vi "禹山pH校准.vi"() -> ()   [LabVIEW 2016, in "斯坦道多参数.lvlib"]
uses:
  <vilib>/Utility/miscctls.llb/LVPointTypeDef.ctl
  <vilib>/Analysis/NI_AALBase.lvlib
  <vilib>/Analysis/NI_AALPro.lvlib
  <vilib>/Utility/config.llb/NI_LVConfig.lvlib
panel:
  out "通讯状态":string
  out "第二点校准值":dbl
  out "第一点校准值":dbl
  out "最小值":sgl format="%.2g"
  out "最大值":sgl format="%.2g"
  in  "校准停止":bool
  in  "校准模式":u16(ring) items=["两点校准", "单点校准"]
  in  "标液2":dbl
  in  "标液1":dbl
  out "波形图表":sgl(graph) caption="历史曲线"
  out "温度测量值":dbl caption="温度" format="%#.2f"
  out "变异系数":dbl format="%.6g"
  out "standard deviation":dbl caption="标准差" format="%0.2f"
  out "mean":dbl caption="均值" format="%0.2f"
  out "提示":string
  in  "校准启动":bool
  out "测试值":dbl format="%#.2f"
  out "电极斜率":dbl format="%#.6f"
  out "电极零点":dbl format="%#.6f"
  # "酸碱度电极设定"
  # "℃"
  # "请选择校准模式:"
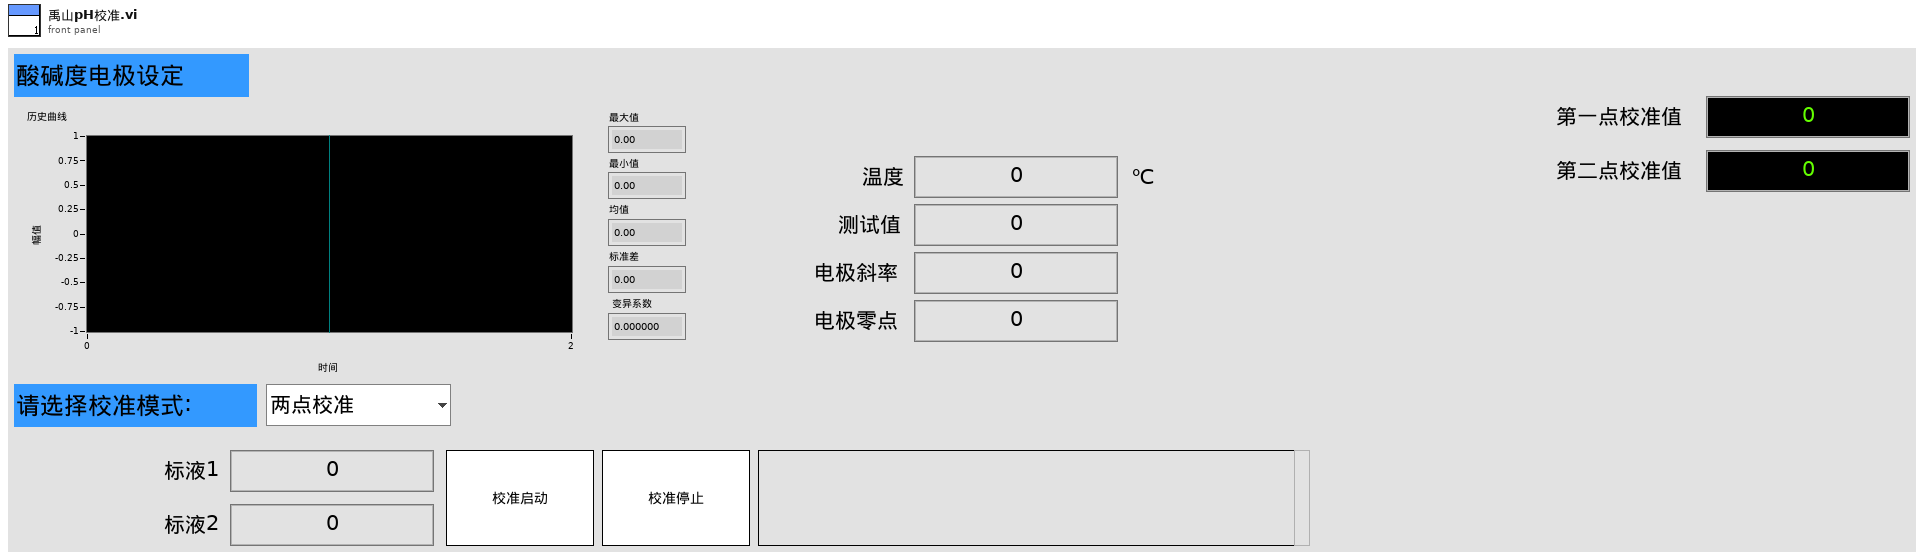
[diagram p1: front panel]
types:
  T1 = typedef "LVPointTypeDef.ctl" = cluster{"Horizontal":i16, "Vertical":i16}
  T2 = typedef "NI_LVConfig.lvlib/Config Data RefNum.ctl" = refnum<k1>
  T3 = enum8{"Enabled", "Disabled", "Disabled and Grayed Out"}
  T4 = cluster{"ph":bool, "DO":bool, "Cond":bool, "Turb":bool, "叶绿素a":bool, "藻密度":bool, "ORP":bool}
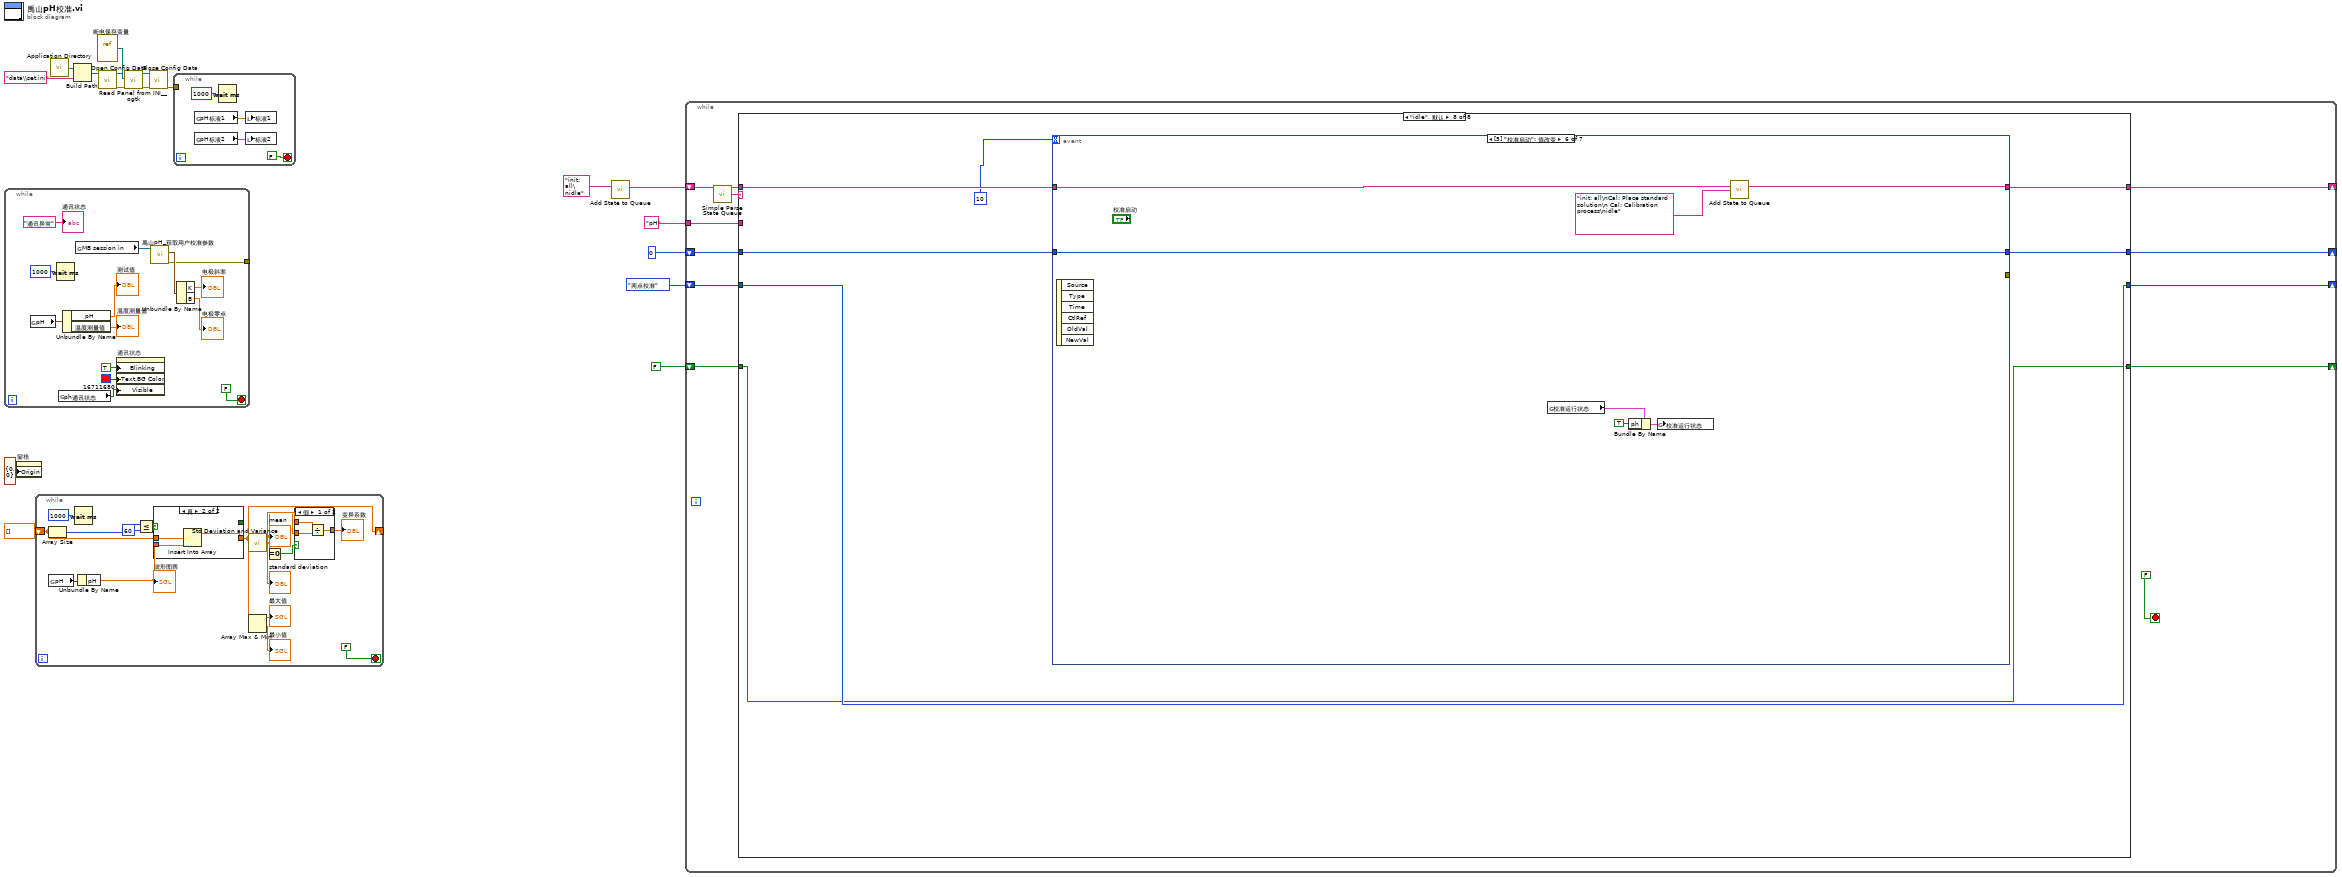
[diagram p0: block diagram]
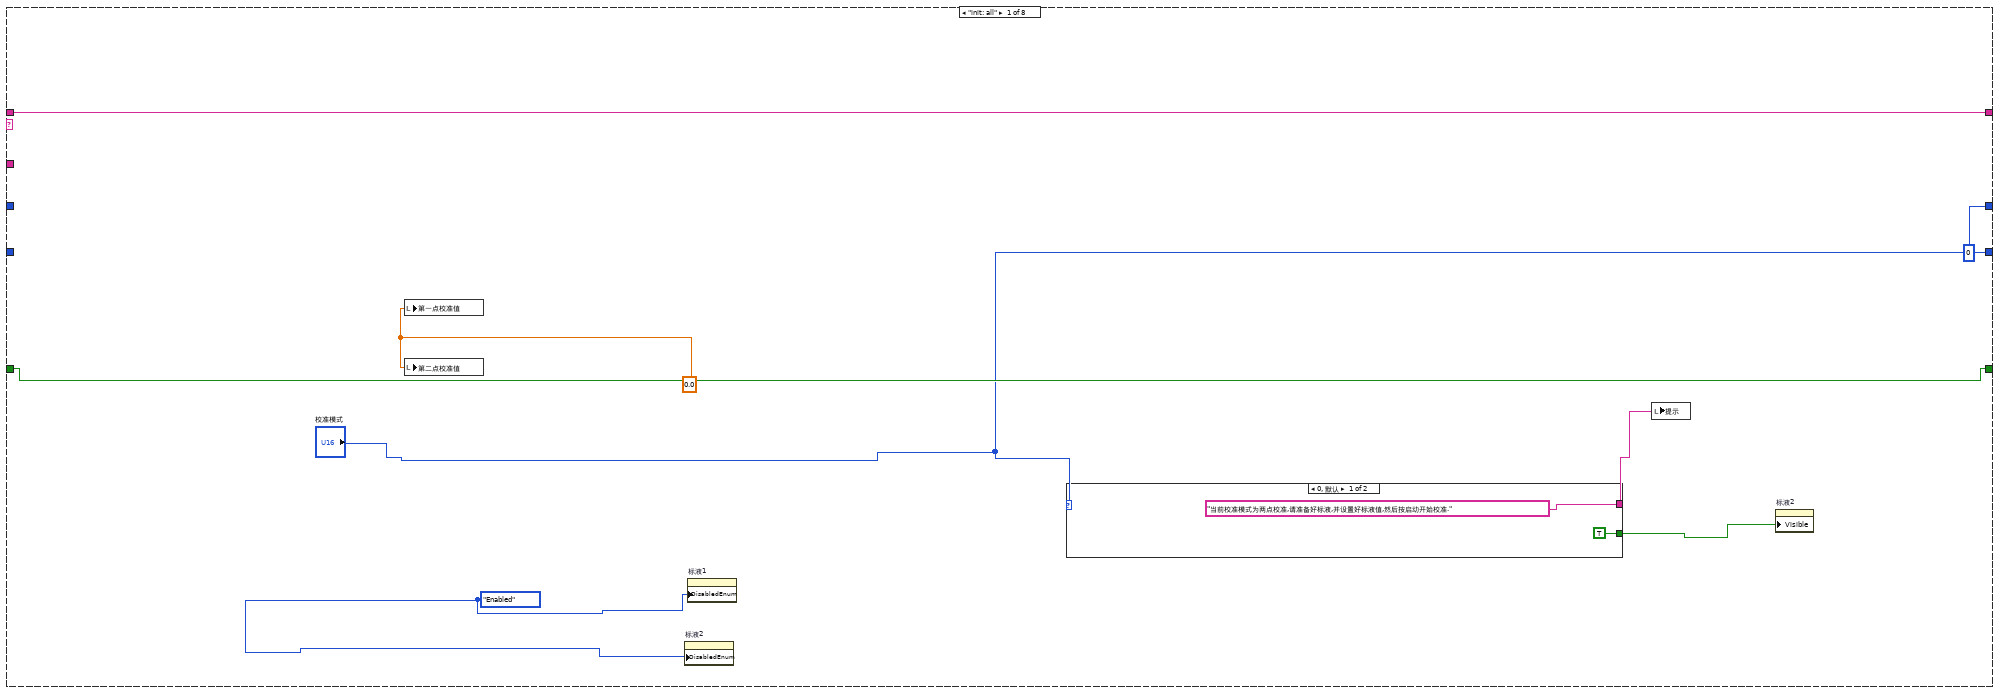
[diagram p2: hidden frame]
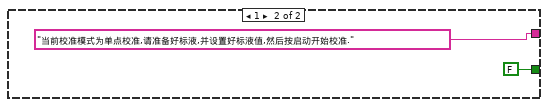
[diagram p3: hidden frame]
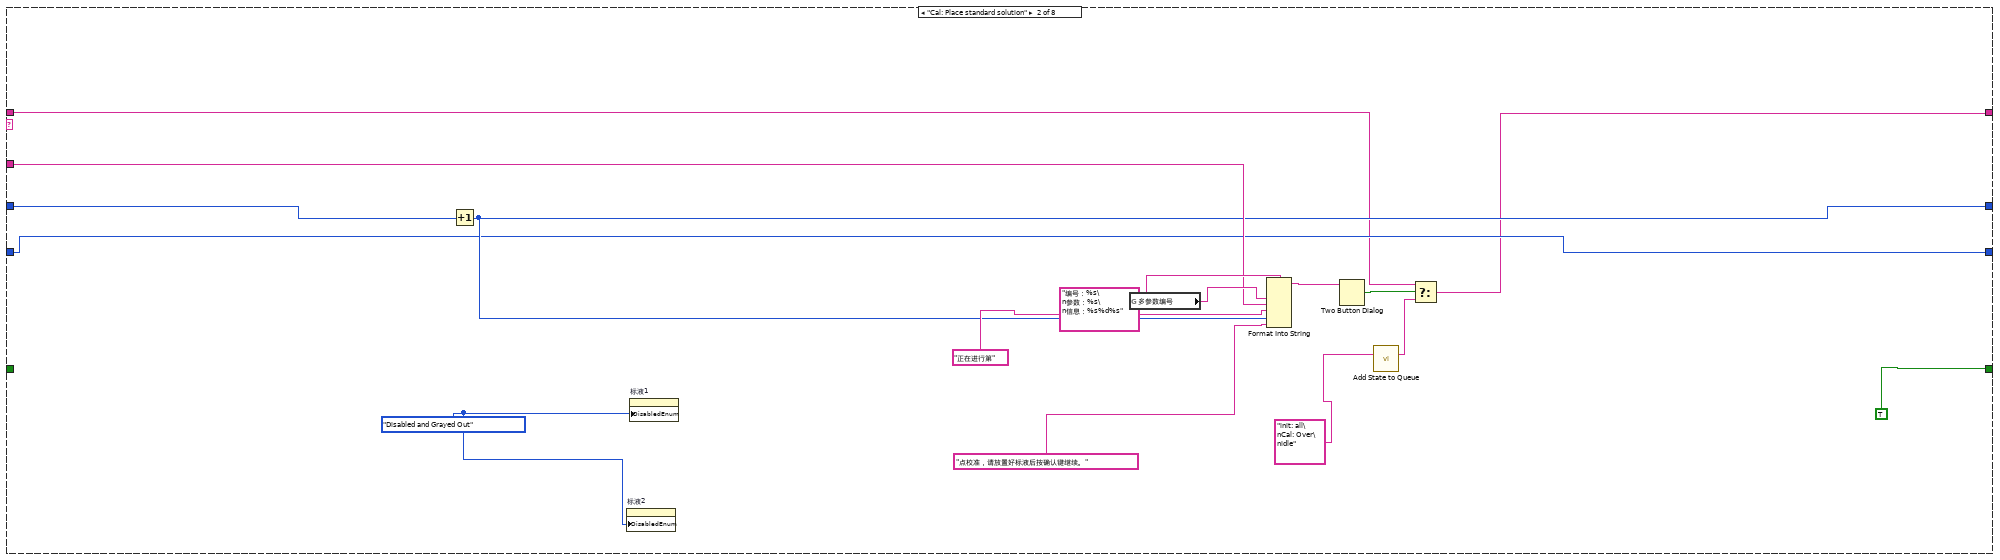
[diagram p4: hidden frame]
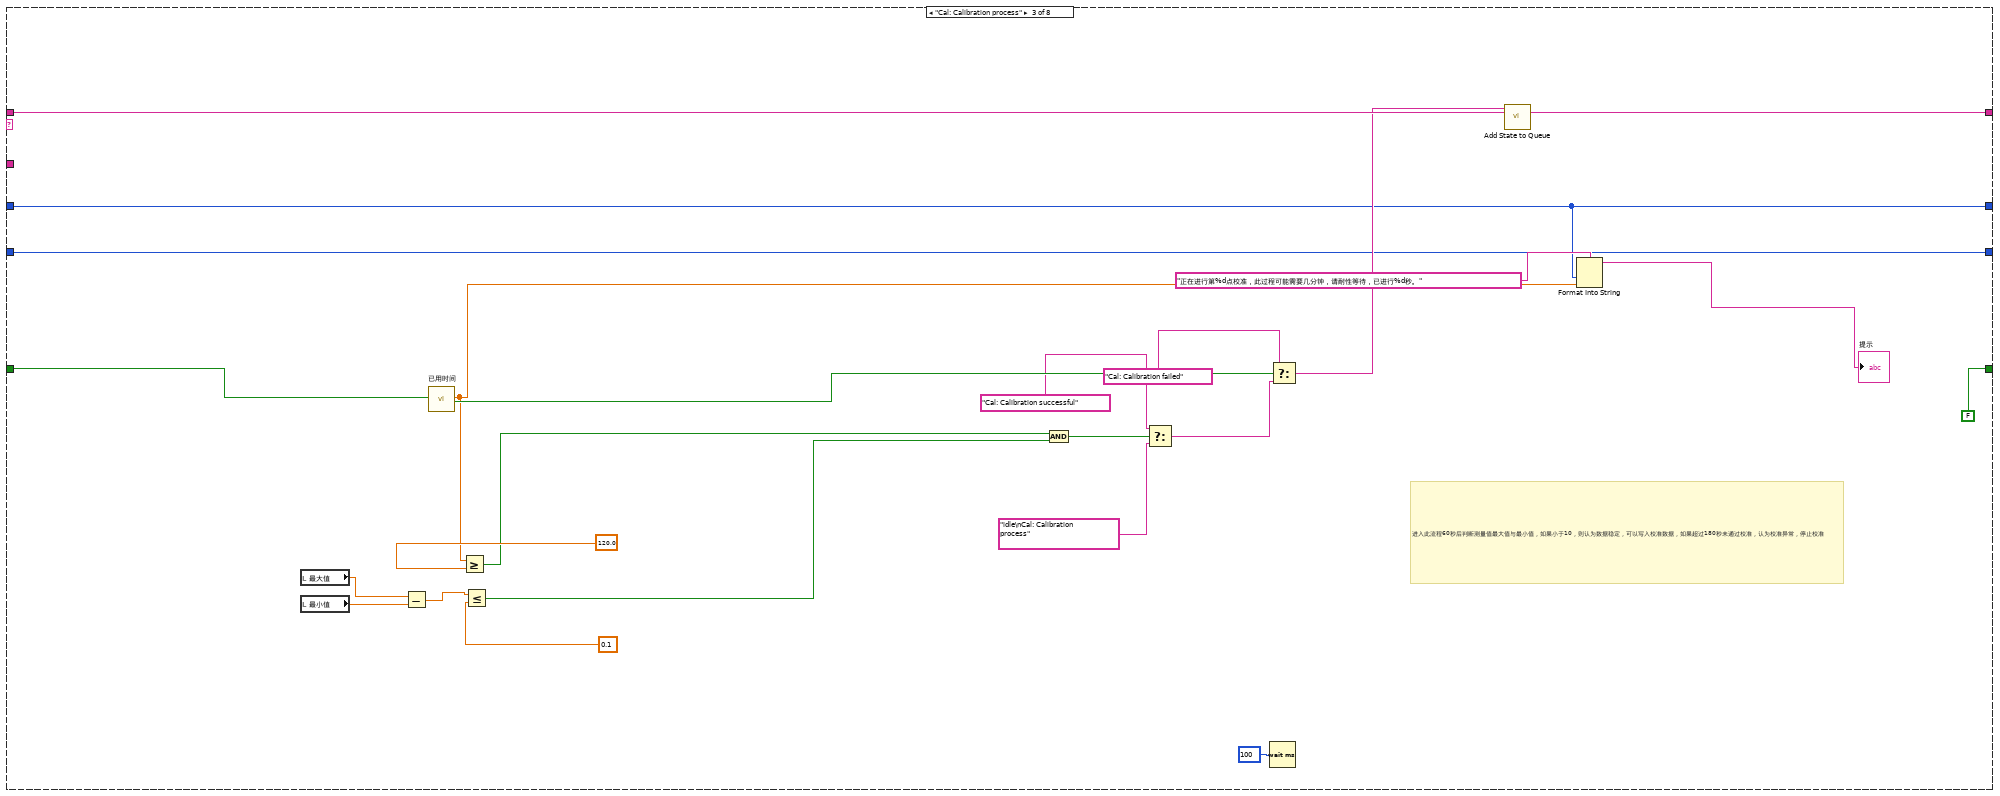
[diagram p5: hidden frame]
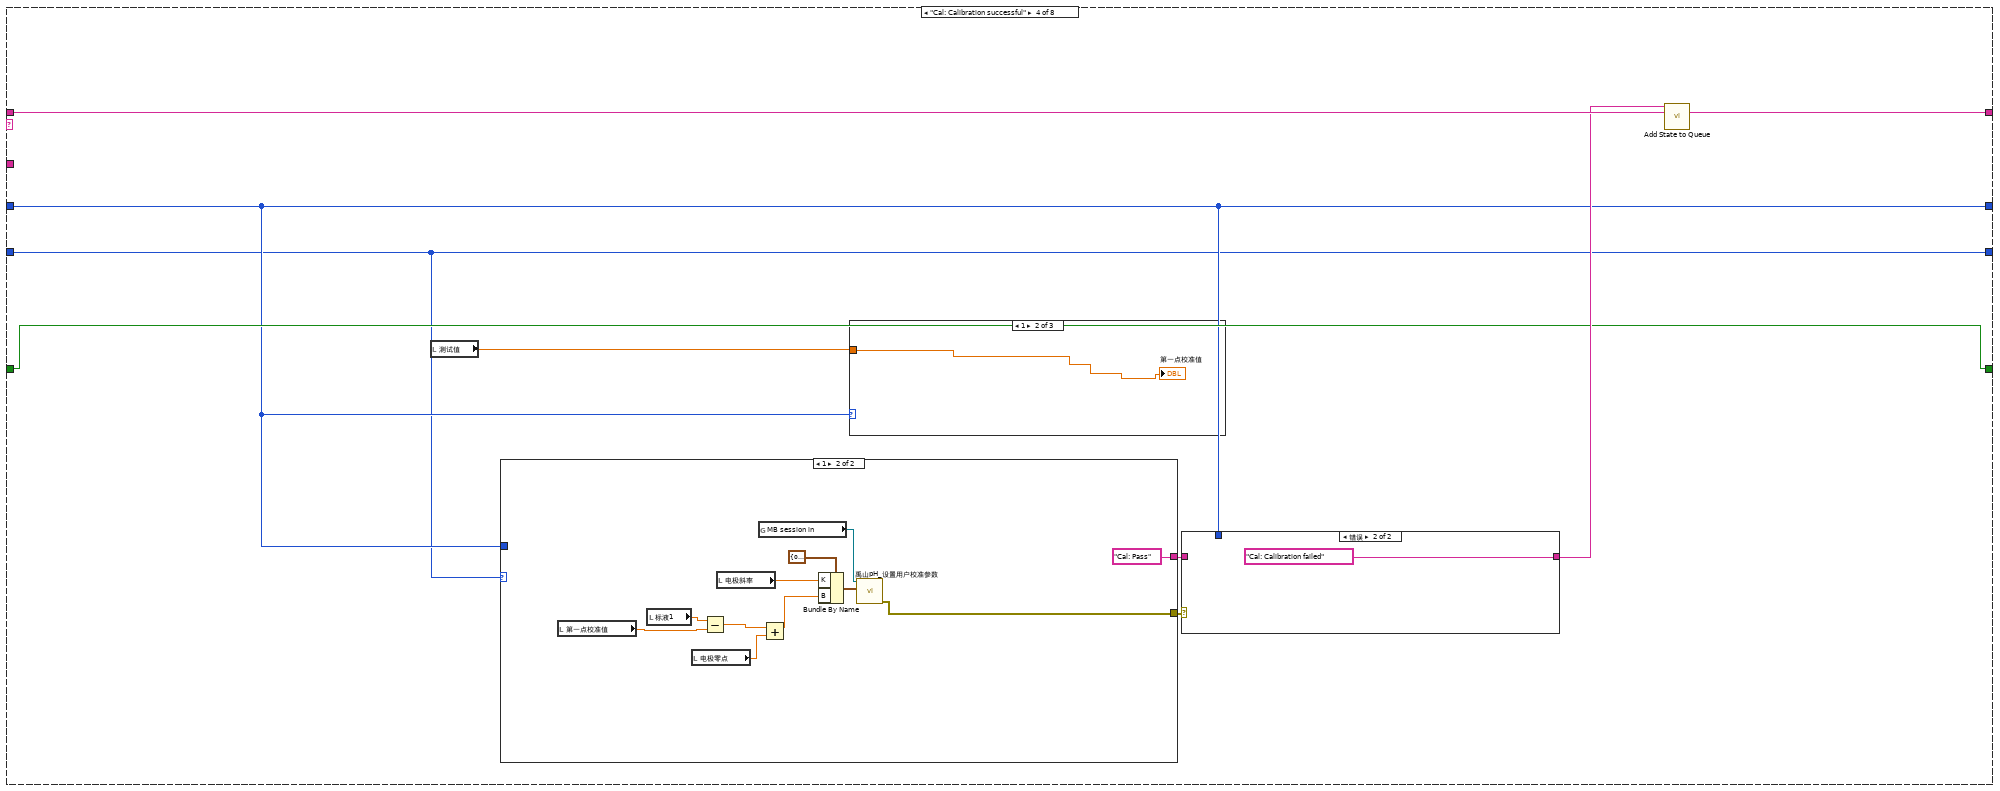
[diagram p6: hidden frame]
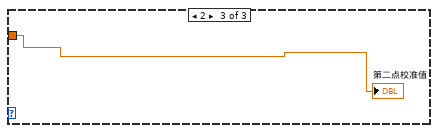
[diagram p8: hidden frame]
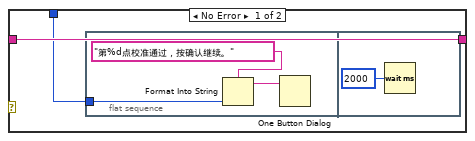
[diagram p9: hidden frame]
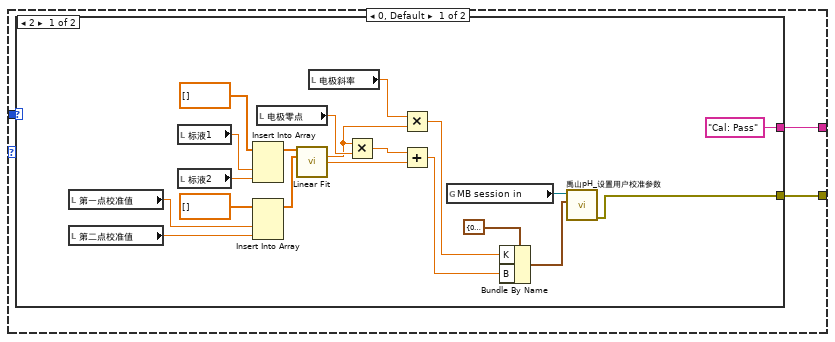
[diagram p10: hidden frame]
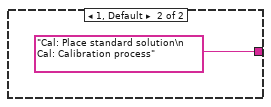
[diagram p11: hidden frame]
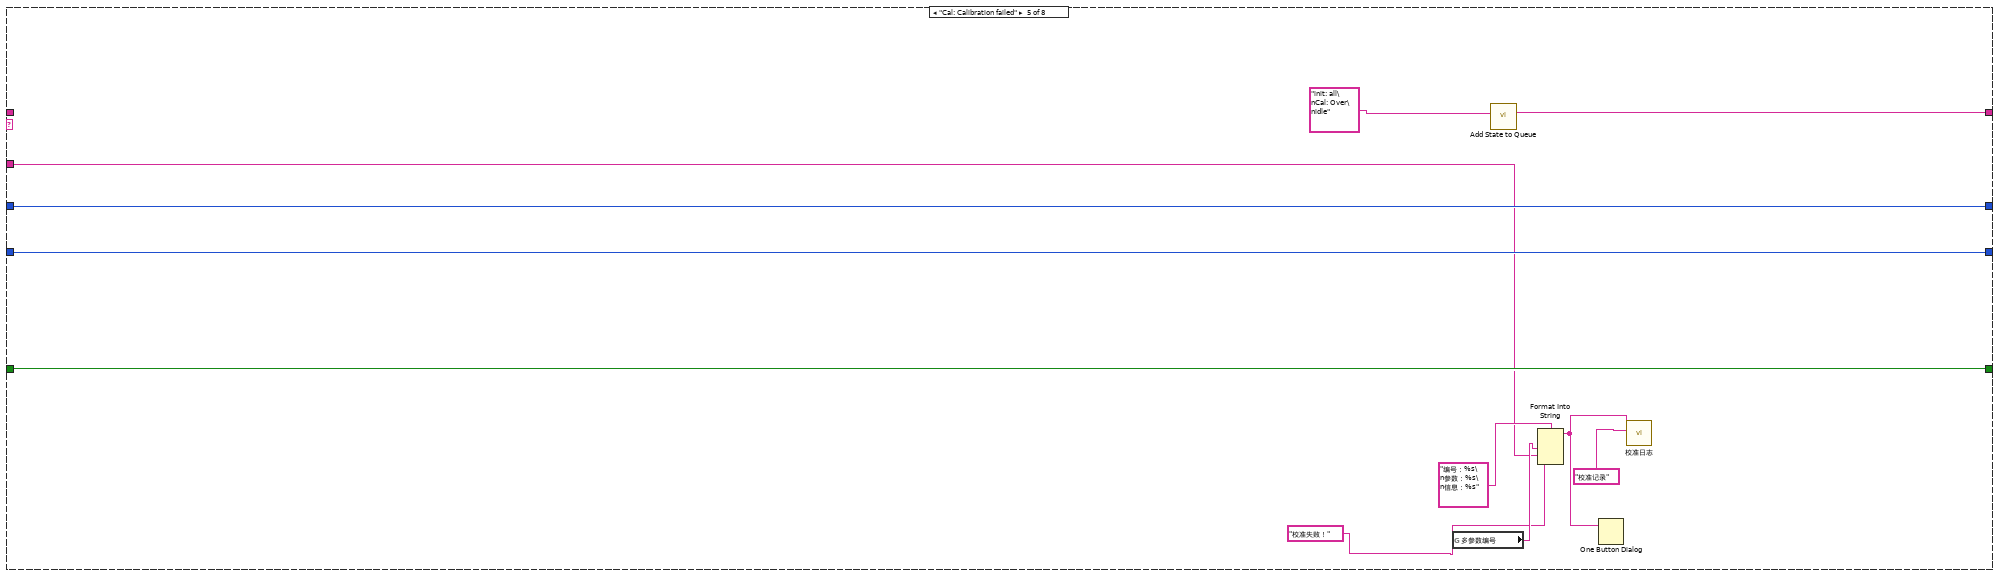
[diagram p12: hidden frame]
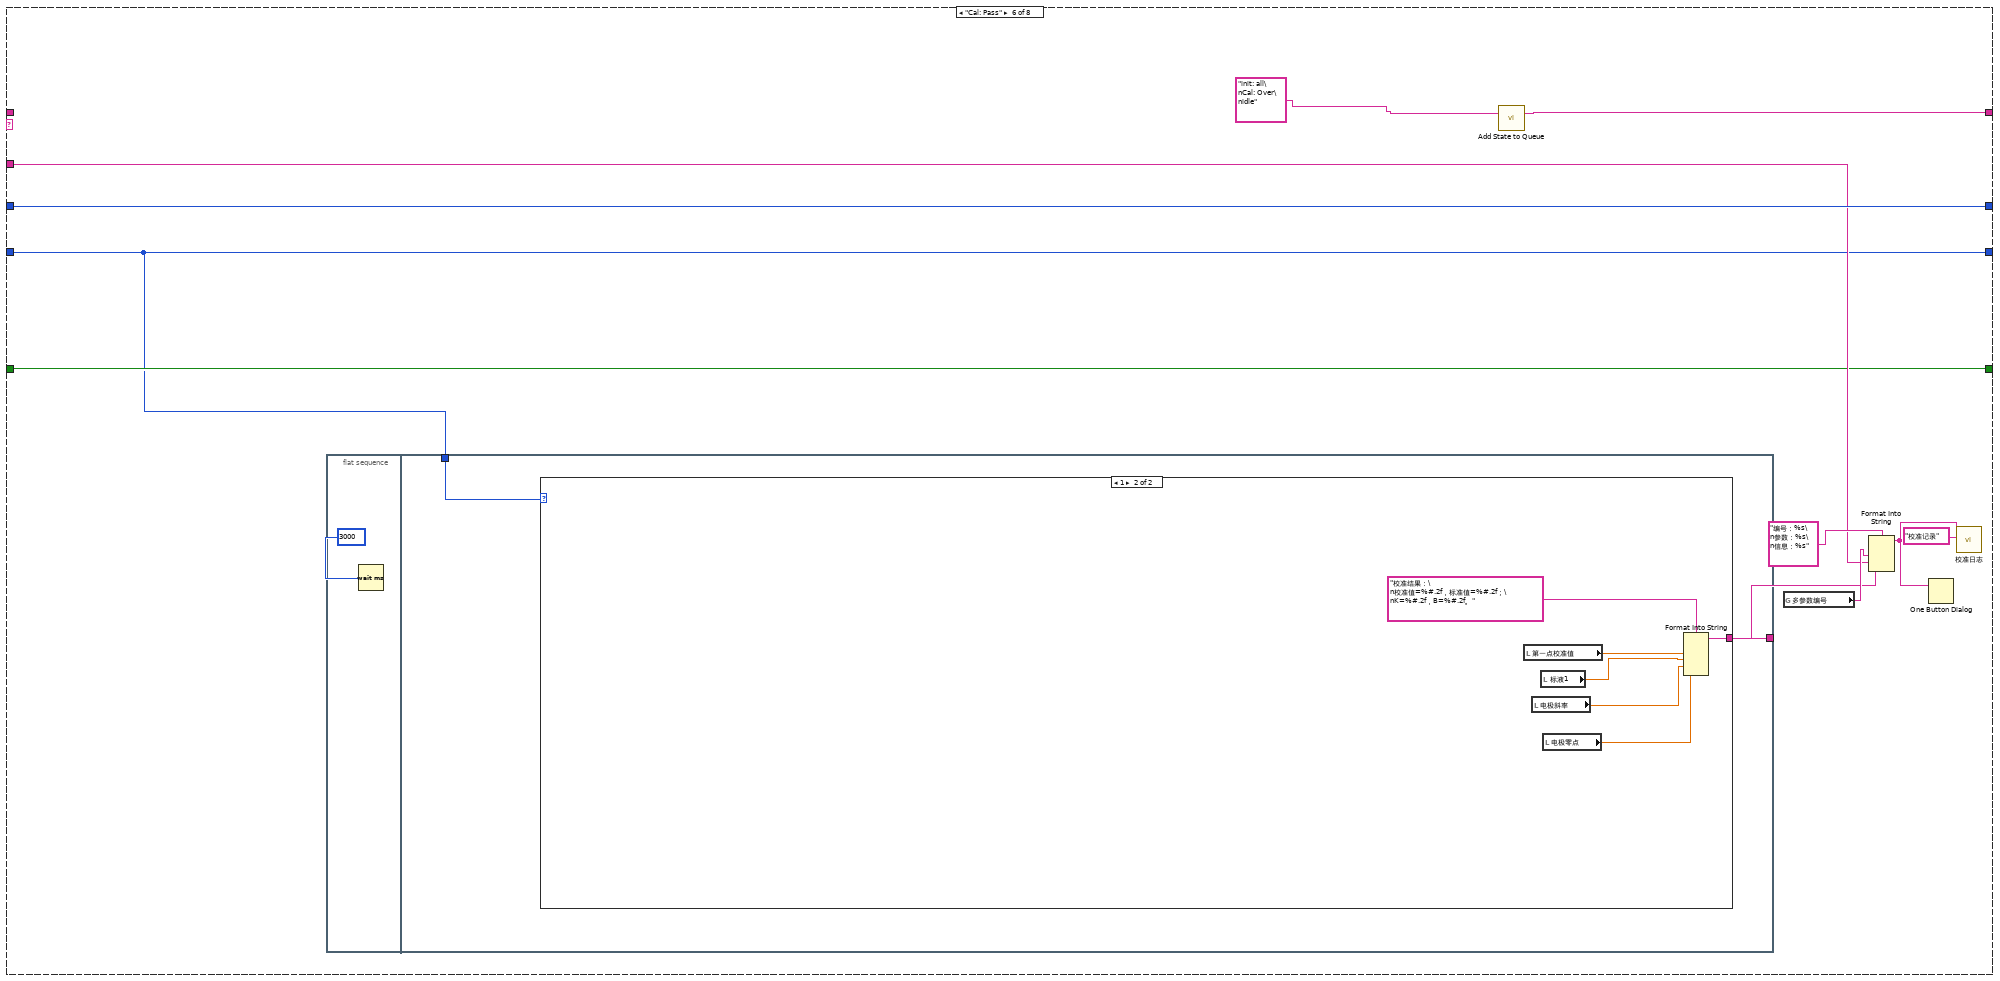
[diagram p13: hidden frame]
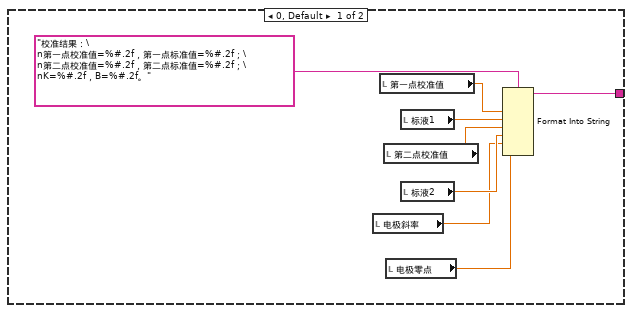
[diagram p14: hidden frame]
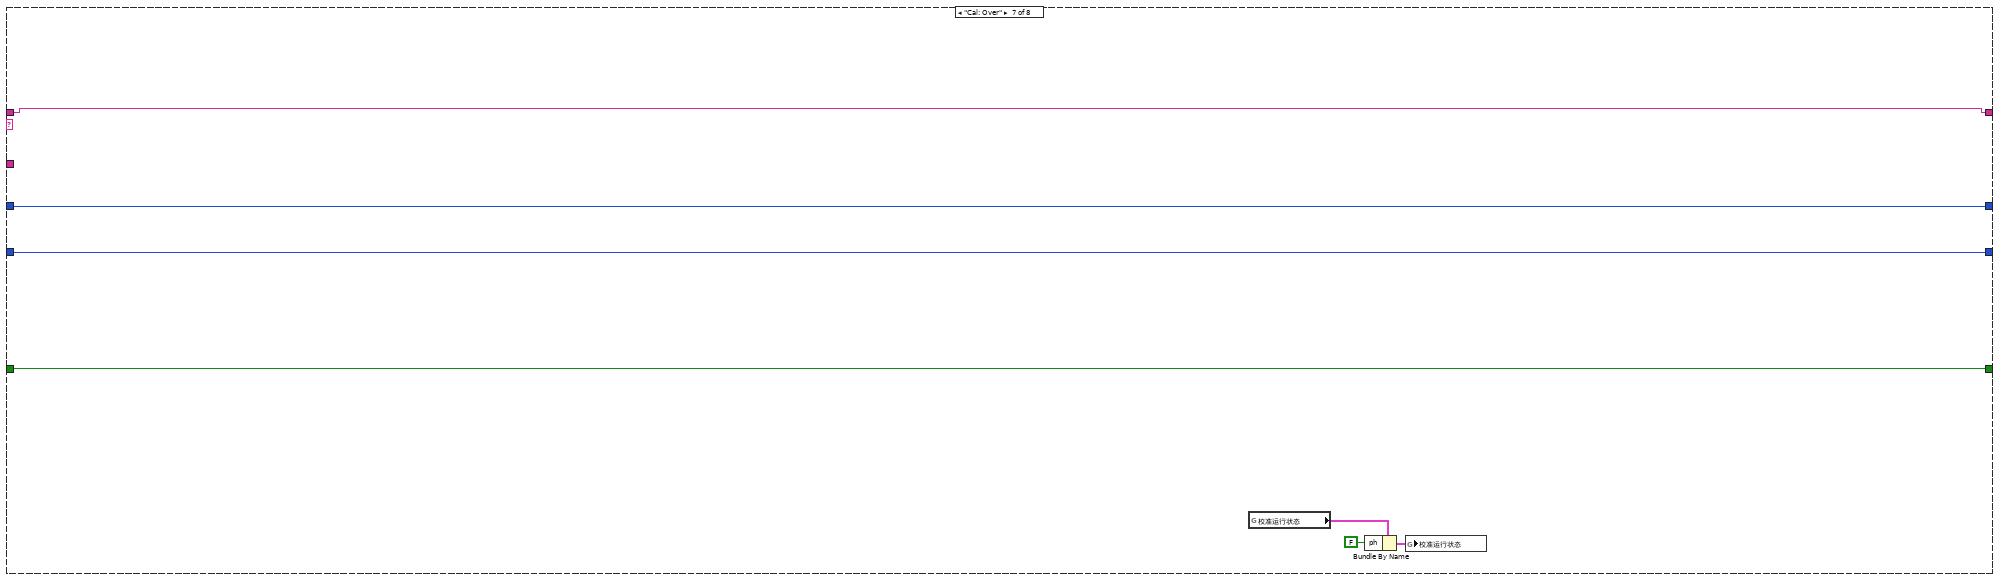
[diagram p15: hidden frame]
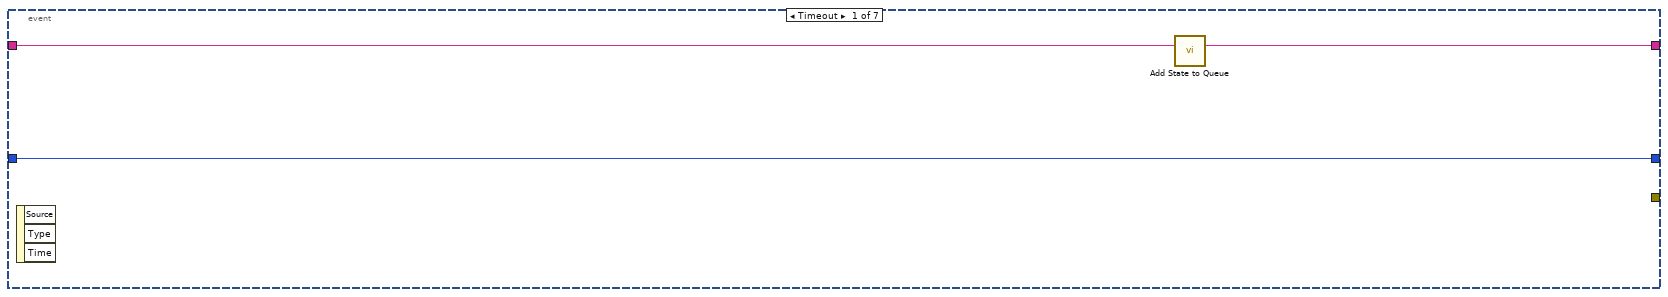
[diagram p16: hidden frame]
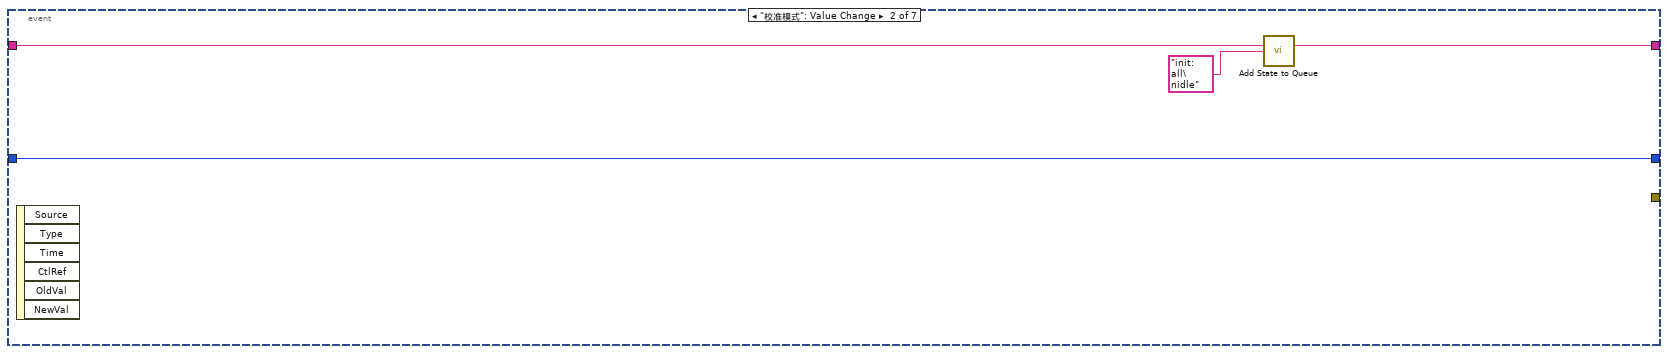
[diagram p17: hidden frame]
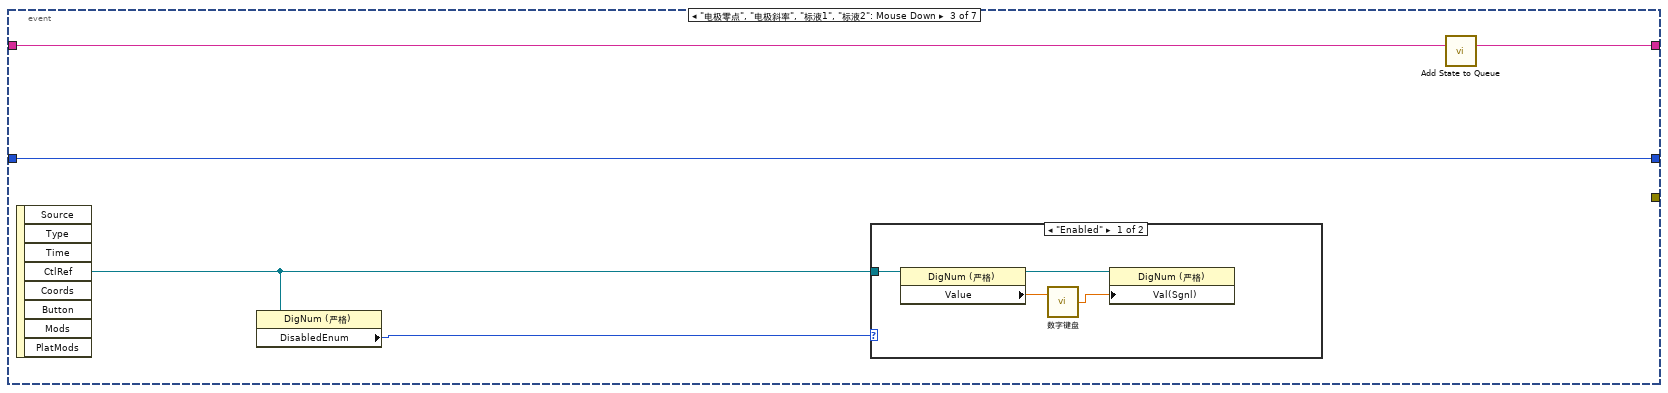
[diagram p18: hidden frame]
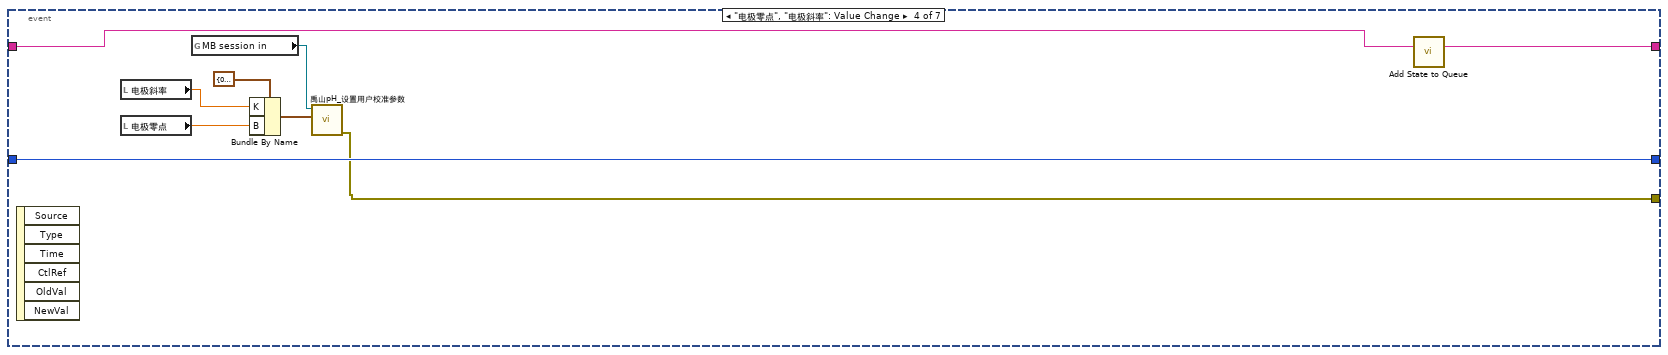
[diagram p20: hidden frame]
diagram:
  n1 = while {
    tunnel: [w26] -> _
    stop <- FALSE stop-if-true
    n2 = global read "禹山过程全局变量.vi" "pH"() -> (w23:cluster{"温度测量值":sgl, "ORP":sgl, "pH":sgl})
    n3 = Wait (ms)(milliseconds to wait=u32 1000 ("等待时间（毫秒）")) -> ()  [unwired: 1 out]
    n4 = global read "多参数全局变量.vi" "ph通讯状态"() -> (w18:bool)
    n5 = Unbundle By Name(w23) -> ("pH"=→"测试值":sgl, "温度测量值"=→"温度测量值":sgl)
    n6 = global read "多参数全局变量.vi" "MB session in"() -> (w22:refnum<class "MB_Master.lvclass">)
    n7 = property on="通讯状态" class="Str"("Blinking"=TRUE ("闪烁"), "Text.BG Color"=u32 16711680, "Visible"=w18) -> ()  [unwired: 2 in, 2 out]
    n8 = call "禹山pH_获取用户校准参数.vi"("MB session in"=w22) -> ("error out"=w26:errorcluster, "输出值"=w29:cluster{"K":sgl, "B":sgl})  [unwired: 8 in, 1 out]
    n9 = Unbundle By Name(w29) -> ("K"=→"电极斜率":sgl, "B"=→"电极零点":sgl)
    "通讯状态" <- "通讯异常" ("当前串口")
  }
  n10 = property on="窗格" class="Pane"("Origin"=T1 {"Horizontal"=0, "Vertical"=0} ("原点")) -> ()  [unwired: 2 in, 2 out]
  n11 = while {
    shift-right: [w35] -> _
    shift-left: sgl[] [] -> [w42]
    stop <- FALSE stop-if-true
    n12 = Array Size(array=w42) -> (size(s)=w44:i32)
    n13 = global read "禹山过程全局变量.vi" "pH"() -> (w36:cluster{"温度测量值":sgl, "ORP":sgl, "pH":sgl})
    n14 = Wait (ms)(milliseconds to wait=u32 1000 ("等待时间（毫秒）")) -> ()  [unwired: 1 out]
    n15 = Unbundle By Name(w36) -> ("pH"=w32:sgl)
    "波形图表" <- w32
    n16 = Less Or Equal?(x=w44, y=60) -> (x <= y?=w43:bool)
    n17 = case shown="真" w43 {
      tunnel: w42 -> [w55 w58]
      tunnel: w32 -> [w53 w57]
      tunnel: [w51 w56] -> w35
      tunnel: [TRUE _] -> _
      frame False {
        n18 = Replace Array Subset(array=w55, new element=w53) -> (w54:sgl[])  [unwired: 1 in]
        n19 = Rotate 1D Array(1:w54, 2:-1 ("n")) -> (0:w51:sgl[])
      }
      frame True {
        n20 = Insert Into Array(array=w58, new element=w57) -> (w56:sgl[])  [unwired: 1 in]
      }
    }
    n21 = call <vilib>:"Std Deviation and Variance.vi"("X"=w35) -> ("mean"=w37:dbl, "standard deviation"=w38:dbl)  [unwired: 1 in, 1 out]
    "standard deviation" <- w38
    "mean" <- w37
    n22 = Array Max & Min(array=w35) -> (max value=→"最大值":sgl, min value=→"最小值":sgl)  [unwired: 2 out]
    n23 = Equal To 0?(x=w37) -> (x = 0?=w41:bool)
    n24 = case shown="假" w41 {
      tunnel: w38 -> [w49 _]
      tunnel: [w48 _] -> w40
      tunnel: w37 -> [w47 _]
      frame False {
        n25 = Divide(x=w49, y=w47) -> (x/y=w48:dbl)
      }
      frame True {
      }
    }
    "变异系数" <- w40
  }
  n26 = call <vilib>:"Application Directory.vi"() -> ("Application Directory"=w12:path)
  n27 = Build Path(base path=w12, name or relative path="data\\set.ini" ("名称或相对路径")) -> (appended path=w13:path)
  n28 = vi-ref "断电保存变量.vi"() -> (w15:refnum<vi>)
  n29 = call <vilib>:"Open Config Data.vi"("configuration file path"=w13) -> ("error out"=w9:errorcluster, "refnum"=w8:T2)  [unwired: 8 in, 1 out]
  n30 = call <userlib>:"Read Panel from INI__ogtk.vi"("error in (no error)"=w9, "VI ref"=w15, "refnum"=w8) -> ("error out"=w11:errorcluster, "refnum out"=w10:T2)  [unwired: 7 in]
  n31 = call <vilib>:"Close Config Data.vi"("error in (no error)"=w11, "refnum"=w10) -> ("error out"=w7:errorcluster)  [unwired: 8 in, 1 out]
  n32 = while {
    tunnel: w7 -> [_]
    stop <- FALSE stop-if-true
    n33 = global read "断电保存变量.vi" "pH标液1"() -> (w60:dbl)
    n34 = global read "断电保存变量.vi" "pH标液2"() -> (w59:dbl)
    n35 = Wait (ms)(milliseconds to wait=u32 1000 ("等待时间（毫秒）")) -> ()  [unwired: 1 out]
    n36 = local write "标液1"(w60) -> ()
    n37 = local write "标液2"(w59) -> ()
  }
  n38 = call "Add State to Queue.vi"("State(s) In (\"\")"="init: all\nidle" ("State(s) In (\"\")")) -> ("States Out"=w5:string)  [unwired: 14 in]
  n39 = while {
    shift-right: [w70] -> _
    shift-left: w5 -> [w74]
    shift-right: [w67] -> _
    shift-left: 0 -> [w69]
    tunnel: "pH" ("State(s) In (\"\")") -> [w68]
    shift-right: [w65] -> _
    shift-left: enum16{"两点校准", "单点校准"}."两点校准" ("校准模式") -> [w66]
    shift-right: [w63] -> _
    shift-left: FALSE -> [w64]
    stop <- FALSE stop-if-true
    n40 = call "Simple Parse State Queue.vi"("State Queue"=w74) -> ("Remain States"=w71:string, "Next State"=w72:string)  [unwired: 13 in]
    n41 = case shown="\"idle\", 默认" w72 {
      tunnel: w71 -> [w82 w90 w121 w133 _ _ w222 w232]
      tunnel: [w82 w89 w120 w132 w187 w192 w222 w231] -> w70
      tunnel: w69 -> [_ w98 w105 w128 w190 w201 w221 w229]
      tunnel: w68 -> [_ w99 _ _ w181 w197 _ _]
      tunnel: [0 w96 w105 w128 w190 w201 w221 w230] -> w67
      tunnel: w66 -> [_ w95 w106 w127 w189 w193 w220 w228]
      tunnel: ["校准模式" w95 w106 w127 w189 w193 w220 w228] -> w65
      tunnel: w64 -> [w79 _ w108 w129 w188 w196 w219 w226]
      tunnel: [w79 TRUE FALSE w129 w188 w196 w219 w226] -> w63
      frame "init: all" {
        w76 = T3."Enabled" ("禁用")
        w78 = 0.0 ("第一点校准值")
        n42 = local write "第一点校准值"(w78) -> ()
        n43 = local write "第二点校准值"(w78) -> ()
        n44 = property on="标液2" class="DigNum (严格)"("DisabledEnum"=w76) -> ()  [unwired: 2 in, 2 out]
        n45 = property on="标液1" class="DigNum (严格)"("DisabledEnum"=w76) -> ()  [unwired: 2 in, 2 out]
        n46 = case shown="0, 默认" "校准模式" {
          tunnel: ["当前校准模式为两点校准,请准备好标液,并设置好标液值,然后按启动开始校准." ("提示") "当前校准模式为单点校准,请准备好标液,并设置好标液值,然后按启动开始校准." ("提示")] -> w81
          tunnel: [TRUE ("可见") FALSE ("可见")] -> w75
          frame 0, Default {
          }
          frame 1 {
          }
        }
        n47 = local write "提示"(w81) -> ()
        n48 = property on="标液2" class="DigNum (严格)"("Visible"=w75) -> ()  [unwired: 2 in, 2 out]
      }
      frame "Cal: Place standard solution" {
        w88 = T3."Disabled and Grayed Out" ("禁用")
        n49 = Increment(x=w98) -> (x+1=w96:i32)
        n50 = property on="标液2" class="DigNum (严格)"("DisabledEnum"=w88) -> ()  [unwired: 2 in, 2 out]
        n51 = property on="标液1" class="DigNum (严格)"("DisabledEnum"=w88) -> ()  [unwired: 2 in, 2 out]
        n52 = global read "多参数全局变量.vi" "多参数编号"() -> (w101:string)
        n53 = Format Into String(format string="编号：%s\n参数：%s\n信息：%s%d%s" ("格式字符串"), w101, w99, "正在进行第" ("消息"), w96, "点校准，请放置好标液后按确认键继续。" ("消息")) -> (resulting string=w93:string)  [unwired: 2 in, 1 out]
        n54 = Two Button Dialog(message=w93) -> (T button?=w92:bool)  [unwired: 2 in]
        n55 = call "Add State to Queue.vi"("State(s) In (\"\")"="init: all\nCal: Over\nidle" ("State(s) In (\"\")")) -> ("States Out"=w91:string)  [unwired: 14 in]
        n56 = Select(t=w90, s=w92, f=w91) -> (s? t:f=w89:string)
      }
      frame "Cal: Calibration process" {
        # "进入此流程60秒后判断测量值最大值与最小值，如果小于10，则认为数据稳定，可以写入校准数据，如果超过180秒未通过校准，认为校准异常，停止校准"
        n57 = local read "最大值"() -> (w125:sgl)
        n58 = local read "最小值"() -> (w124:sgl)
        n59 = Subtract(x=w125, y=w124) -> (x-y=w126:sgl)
        n60 = call "已用时间"("Reset"=w108) -> ("Elapsed Time (s)"=w104:dbl, "Time has Elapsed"=w122:bool)  [unwired: 11 in, 6 out]
        n61 = Greater Or Equal?(x=w104, y=120.0) -> (x >= y?=w117:bool)
        n62 = Less Or Equal?(x=w126, y=0.1) -> (x <= y?=w113:bool)
        n63 = And(x=w117, y=w113) -> (x .and. y?=w114:bool)
        n64 = Select(t="Cal: Calibration successful" ("State(s) In (\"\")"), s=w114, f="idle\nCal: Calibration process" ("State(s) In (\"\")")) -> (s? t:f=w112:string)
        n65 = Wait (ms)(milliseconds to wait=u32 100 ("等待时间（毫秒）")) -> ()  [unwired: 1 out]
        n66 = Select(t="Cal: Calibration failed" ("State(s) In (\"\")"), s=w122, f=w112) -> (s? t:f=w111:string)
        n67 = call "Add State to Queue.vi"("State(s) In Front (\"\")"=w111, "State(s) In (\"\")"=w121) -> ("States Out"=w120:string)  [unwired: 13 in]
        n68 = Format Into String(format string="正在进行第%d点校准，此过程可能需要几分钟，请耐性等待，已进行%d秒。" ("格式字符串"), w105, w104) -> (resulting string=→"提示":string)  [unwired: 2 in, 1 out]
      }
      frame "Cal: Calibration successful" {
        n69 = local read "测试值"() -> (w130:dbl)
        n70 = case shown="1" w127 {
          tunnel: [w147 w169] -> w135
          tunnel: [w146 "Cal: Pass" ("State(s) In (\"\")")] -> w134
          tunnel: w128 -> [w145 _]
          frame 0, Default {
            n71 = case shown="2" w145 {
              tunnel: [w148 _] -> w147
              tunnel: ["Cal: Pass" ("State(s) In (\"\")") "Cal: Place standard solution\n Cal: Calibration process" ("State(s) In (\"\")")] -> w146
              frame 2 {
                n72 = local read "第一点校准值"() -> (w150:dbl)
                n73 = local read "第二点校准值"() -> (w151:dbl)
                n74 = local read "标液1"() -> (w153:dbl)
                n75 = local read "标液2"() -> (w154:dbl)
                n76 = Insert Into Array(array=dbl[] [] ("Weight"), new element #1=w153, new element #2=w154) -> (w155:dbl[])  [unwired: 1 in]
                n77 = Insert Into Array(array=dbl[] [] ("Weight"), new element #1=w150, new element #2=w151) -> (w156:dbl[])  [unwired: 1 in]
                n78 = local read "电极零点"() -> (w163:dbl)
                n79 = call <vilib>:"Linear Fit.vi"("Y"=w155, "X"=w156) -> ("slope"=w162:dbl, "intercept"=w165:dbl)  [unwired: 9 in, 3 out]
                n80 = local read "电极斜率"() -> (w160:dbl)
                n81 = Multiply(x=w162, y=w163) -> (x*y=w164:dbl)
                n82 = Multiply(x=w160, y=w162) -> (x*y=w161:dbl)
                n83 = Add(x=w164, y=w165) -> (x+y=w166:dbl)
                n84 = global read "多参数全局变量.vi" "MB session in"() -> (w157:refnum<class "MB_Master.lvclass">)
                n85 = Bundle By Name(cluster=cluster{"K":sgl, "B":sgl} {"K"=0.0, "B"=0.0} ("用户校准参数"), "K"=w161, "B"=w166) -> (w158:cluster{"K":sgl, "B":sgl})
                n86 = call "禹山pH_设置用户校准参数.vi"("用户校准参数"=w158, "MB session in"=w157) -> ("error out"=w148:errorcluster)  [unwired: 8 in, 1 out]
              }
              frame 1, Default {
              }
            }
          }
          frame 1 {
            n87 = local read "第一点校准值"() -> (w174:dbl)
            n88 = local read "标液1"() -> (w175:dbl)
            n89 = local read "电极零点"() -> (w178:dbl)
            n90 = Subtract(x=w175, y=w174) -> (x-y=w176:dbl)
            n91 = local read "电极斜率"() -> (w170:dbl)
            n92 = global read "多参数全局变量.vi" "MB session in"() -> (w171:refnum<class "MB_Master.lvclass">)
            n93 = Add(x=w176, y=w178) -> (x+y=w177:dbl)
            n94 = Bundle By Name(cluster=cluster{"K":sgl, "B":sgl} {"K"=0.0, "B"=0.0} ("用户校准参数"), "K"=w170, "B"=w177) -> (w172:cluster{"K":sgl, "B":sgl})
            n95 = call "禹山pH_设置用户校准参数.vi"("用户校准参数"=w172, "MB session in"=w171) -> ("error out"=w169:errorcluster)  [unwired: 8 in, 1 out]
          }
        }
        n96 = case shown="1" w128 {
          tunnel: w130 -> [_ w136 w137]
          frame 0, Default {
          }
          frame 1 {
            "第一点校准值" <- w136
          }
          frame 2 {
            "第二点校准值" <- w137
          }
        }
        n97 = case shown="错误" w135 {
          tunnel: w134 -> [w139 _]
          tunnel: [w139 "Cal: Calibration failed" ("State(s) In (\"\")")] -> w131
          tunnel: w128 -> [w138 _]
          frame No Error {
            n98 = flat-sequence {
              tunnel: w138 -> [w140]
              frame #0 {
                n99 = Format Into String(format string="第%d点校准通过，按确认继续。" ("格式字符串"), w140) -> (resulting string=w142:string)  [unwired: 2 in, 1 out]
                n100 = One Button Dialog(message=w142) -> ()  [unwired: 1 in, 1 out]
              }
              frame #1 {
                n101 = Wait (ms)(milliseconds to wait=u32 2000 ("等待时间（毫秒）")) -> ()  [unwired: 1 out]
              }
            }
          }
          frame Error {
          }
        }
        n102 = call "Add State to Queue.vi"("State(s) In Front (\"\")"=w131, "State(s) In (\"\")"=w133) -> ("States Out"=w132:string)  [unwired: 13 in]
      }
      frame "Cal: Calibration failed" {
        n103 = global read "多参数全局变量.vi" "多参数编号"() -> (w184:string)
        n104 = call "Add State to Queue.vi"("State(s) In (\"\")"="init: all\nCal: Over\nidle" ("State(s) In (\"\")")) -> ("States Out"=w187:string)  [unwired: 14 in]
        n105 = Format Into String(format string="编号：%s\n参数：%s\n信息：%s" ("格式字符串"), w184, w181, "校准失败！" ("消息")) -> (resulting string=w183:string)  [unwired: 2 in, 1 out]
        n106 = One Button Dialog(message=w183) -> ()  [unwired: 1 in, 1 out]
        n107 = call "校准日志.vi"("table"="校准记录", "日志信息"=w183) -> ()  [unwired: 9 in, 1 out]
      }
      frame "Cal: Pass" {
        n108 = flat-sequence {
          tunnel: [w204] -> w194
          tunnel: w193 -> [w203]
          frame #0 {
            n109 = Wait (ms)(milliseconds to wait=u32 3000 ("等待时间（毫秒）")) -> ()  [unwired: 1 out]
          }
          frame #1 {
            n110 = case shown="1" w203 {
              tunnel: [w212 w218] -> w204
              frame 0, Default {
                n111 = local read "电极斜率"() -> (w206:dbl)
                n112 = local read "第一点校准值"() -> (w210:dbl)
                n113 = local read "第二点校准值"() -> (w208:dbl)
                n114 = local read "电极零点"() -> (w205:dbl)
                n115 = local read "标液1"() -> (w211:dbl)
                n116 = local read "标液2"() -> (w207:dbl)
                n117 = Format Into String(format string="校准结果：\n第一点校准值=%#.2f，第一点标准值=%#.2f；\n第二点校准值=%#.2f，第二点标准值=%#.2f；\nK=%#.2f，B=%#.2f。" ("提示"), w210, w211, w208, w207, w206, w205) -> (resulting string=w212:string)  [unwired: 2 in, 1 out]
              }
              frame 1 {
                n118 = local read "第一点校准值"() -> (w217:dbl)
                n119 = local read "电极斜率"() -> (w214:dbl)
                n120 = local read "标液1"() -> (w215:dbl)
                n121 = local read "电极零点"() -> (w213:dbl)
                n122 = Format Into String(format string="校准结果：\n校准值=%#.2f，标准值=%#.2f；\nK=%#.2f，B=%#.2f。" ("提示"), w217, w215, w214, w213) -> (resulting string=w218:string)  [unwired: 2 in, 1 out]
              }
            }
          }
        }
        n123 = call "Add State to Queue.vi"("State(s) In (\"\")"="init: all\nCal: Over\nidle" ("State(s) In (\"\")")) -> ("States Out"=w192:string)  [unwired: 14 in]
        n124 = global read "多参数全局变量.vi" "多参数编号"() -> (w198:string)
        n125 = Format Into String(format string="编号：%s\n参数：%s\n信息：%s" ("格式字符串"), w198, w197, w194) -> (resulting string=w195:string)  [unwired: 2 in, 1 out]
        n126 = One Button Dialog(message=w195) -> ()  [unwired: 1 in, 1 out]
        n127 = call "校准日志.vi"("table"="校准记录", "日志信息"=w195) -> ()  [unwired: 9 in, 1 out]
      }
      frame "Cal: Over" {
        n128 = global read "多参数全局变量.vi" "校准运行状态"() -> (w224:T4)
        n129 = Bundle By Name(cluster=w224, "ph"=FALSE) -> (w225:T4)
        n130 = global write "多参数全局变量.vi" "校准运行状态"(w225) -> ()
      }
      frame "idle", Default {
        n131 = event shown="[5] \"校准启动\": 值改变" {
          selector: _ -> [_ _ _ _ _ _ _]
          dyn-events: _ -> [_ _ _ _ _ _ _]
          timeout: 10 -> [_ _ _ _ _ _ _]
          tunnel: [_ _ _ w250 _ _ _] -> _
          tunnel: w232 -> [w235 w239 w242 w249 w258 w283 _]
          tunnel: [w234 w238 w243 w256 w259 w282 w285] -> w231
          tunnel: [w233 w236 w244 w257 w260 w280 w286] -> w230
          tunnel: w229 -> [w233 w236 w244 w257 w260 w280 w286]
          event Timeout {
            n132 = event-data() -> ()  [unwired: 1 in, 3 out]
            n133 = call "Add State to Queue.vi"("State(s) In (\"\")"=w235) -> ("States Out"=w234:string)  [unwired: 14 in]
          }
          event "校准模式": Value Change {
            n134 = event-data() -> ()  [unwired: 1 in, 6 out]
            n135 = call "Add State to Queue.vi"("State(s) In (\"\")"=w239, "State(s) At Back (\"\")"="init: all\nidle" ("State(s) In (\"\")")) -> ("States Out"=w238:string)  [unwired: 13 in]
          }
          event "电极零点", "电极斜率", "标液1", "标液2": Mouse Down {
            n136 = event-data() -> ("CtlRef"=w241:refnum<vi>)  [unwired: 1 in, 7 out]
            n137 = property class="DigNum (严格)"(reference=w241) -> ("DisabledEnum"=w240:T3)  [unwired: 1 in, 2 out]
            n138 = case shown="\"Enabled\"" w240 {
              tunnel: w241 -> [w248 _]
              frame "Enabled" {
                n139 = property class="DigNum (严格)"(reference=w248) -> (reference out=w245:refnum<vi>, "Value"=w246:dbl)  [unwired: 1 in, 1 out]
                n140 = call "数字键盘.vi"("OldNumber"=w246) -> ("NewNumber"=w247:dbl)  [unwired: 1 in]
                n141 = property class="DigNum (严格)"(reference=w245, "Val(Sgnl)"=w247) -> ()  [unwired: 1 in, 2 out]
              }
              frame "Disabled", Default {
              }
            }
            n142 = call "Add State to Queue.vi"("State(s) In (\"\")"=w242) -> ("States Out"=w243:string)  [unwired: 14 in]
          }
          event "电极零点", "电极斜率": Value Change {
            n143 = event-data() -> ()  [unwired: 1 in, 6 out]
            n144 = local read "电极斜率"() -> (w253:dbl)
            n145 = local read "电极零点"() -> (w254:dbl)
            n146 = global read "多参数全局变量.vi" "MB session in"() -> (w255:refnum<class "MB_Master.lvclass">)
            n147 = Bundle By Name(cluster=cluster{"K":sgl, "B":sgl} {"K"=0.0, "B"=0.0} ("用户校准参数"), "K"=w253, "B"=w254) -> (w252:cluster{"K":sgl, "B":sgl})
            n148 = call "禹山pH_设置用户校准参数.vi"("用户校准参数"=w252, "MB session in"=w255) -> ("error out"=w250:errorcluster)  [unwired: 8 in, 1 out]
            n149 = call "Add State to Queue.vi"("State(s) In (\"\")"=w249) -> ("States Out"=w256:string)  [unwired: 14 in]
          }
          event "标液1", "标液2": Value Change {
            n150 = event-data() -> ()  [unwired: 1 in, 6 out]
            n151 = flat-sequence {
              frame #0 {
                n152 = global write "断电保存变量.vi" "pH标液1"("标液1") -> ()
                n153 = global write "断电保存变量.vi" "pH标液2"("标液2") -> ()
              }
              frame #1 {
                n154 = call <vilib>:"Application Directory.vi"() -> ("Application Directory"=w272:path)
                n155 = Build Path(base path=w272, name or relative path="data\\set.ini" ("名称或相对路径")) -> (appended path=w271:path)
                n156 = call <vilib>:"Open Config Data.vi"("configuration file path"=w271) -> ("error out"=w275:errorcluster, "refnum"=w276:T2)  [unwired: 8 in, 1 out]
                n157 = vi-ref "断电保存变量.vi"() -> (w269:refnum<vi>)
                n158 = call <userlib>:"Write Panel to INI__ogtk.vi"("error in (no error)"=w275, "VI ref"=w269, "refnum"=w276) -> ("error out"=w273:errorcluster, "refnum out"=w274:T2)  [unwired: 7 in]
                n159 = call <vilib>:"Close Config Data.vi"("error in (no error)"=w273, "refnum"=w274) -> ("error out"=w265:errorcluster, "file path"=w266:path)  [unwired: 8 in]
                n160 = Open/Create/Replace File(file path (use dialog)=w266, error in=w265) -> (refnum out=w267:refnum<file>, error out=w268:errorcluster)  [unwired: 4 in, 1 out]
                n161 = Flush File(refnum=w267, error in=w268) -> (refnum out=w263:refnum<file>, error out=w264:errorcluster)
                n162 = Close File(refnum=w263, error in=w264) -> ()  [unwired: 2 out]
              }
            }
            n163 = call "Add State to Queue.vi"("State(s) In (\"\")"=w258) -> ("States Out"=w259:string)  [unwired: 14 in]
          }
          event "校准启动": Value Change {
            n164 = event-data() -> ()  [unwired: 1 in, 6 out]
            n165 = global read "多参数全局变量.vi" "校准运行状态"() -> (w278:T4)
            n166 = Bundle By Name(cluster=w278, "ph"=TRUE) -> (w279:T4)
            n167 = global write "多参数全局变量.vi" "校准运行状态"(w279) -> ()
            n168 = call "Add State to Queue.vi"("State(s) In (\"\")"=w283, "State(s) At Back (\"\")"="init: all\nCal: Place standard solution\n Cal: Calibration process\nidle" ("State(s) In (\"\")")) -> ("States Out"=w282:string)  [unwired: 13 in]
          }
          event "校准停止": Value Change {
            n169 = event-data() -> ()  [unwired: 1 in, 6 out]
            n170 = call "Add State to Queue.vi"("State(s) In (\"\")"="init: all\nCal: Over\nidle" ("State(s) In (\"\")")) -> ("States Out"=w285:string)  [unwired: 14 in]
          }
        }
      }
    }
  }
